vi "Read URI.vi"(8 "error in (no error)":errorcluster, 11 "WebSocket Server in":refnum<class "WebSocket Server.lvclass">) -> (0 "error out":errorcluster, 2 "URI":string, 3 "WebSocket Server out":refnum<class "WebSocket Server.lvclass">)   [LabVIEW 2016, in "WebSocket Actors.lvlib" / "WebSocket Server.lvclass"]
uses:
  WebSocket Server.lvclass
  WebSocket Server.lvclass/WebSocket Server.ctl
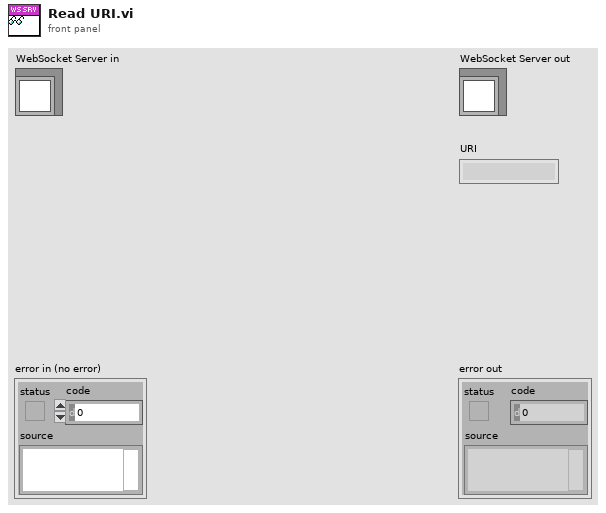
[diagram p1: front panel]
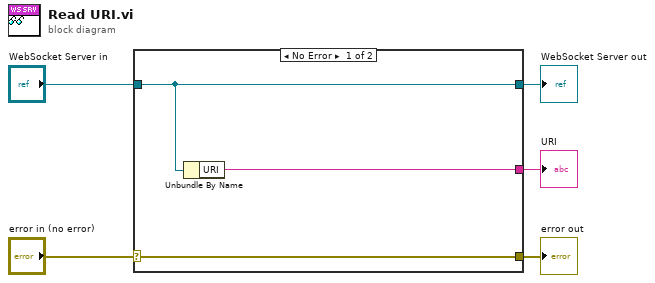
[diagram p0: block diagram]
diagram:
  n1 = case shown="No Error" "error in (no error)" {
    selector: "error in (no error)" -> [w8 w9]
    tunnel: [w8 w9] -> w4
    tunnel: [w7 w10] -> w2
    tunnel: "WebSocket Server in" -> [w7 w10]
    tunnel: [w6 _] -> w1
    frame No Error {
      n2 = Unbundle By Name(w7) -> ("URI"=w6:string)
    }
    frame Error {
    }
  }
  "error out" <- w4
  "WebSocket Server out" <- w2
  "URI" <- w1
